vi "_Get Measurement.vi"(8 "error in (no error)":errorcluster, 10 "Command":string, 11 "VISA resource name":refnum<visa-resource-name>) -> (0 "error out":errorcluster, 1 "Data":dbl[](array[numeric]) format="%^.3e", 2 "Reliability":i32, 3 "VISA resource name out":refnum<visa-resource-name>)   [LabVIEW 2020, in "Rohde&Schwarz CMXP GPRF.lvlib"]
uses:
  <instrlib>/Rohde&Schwarz CMXP GPRF/Rohde&Schwarz CMXP GPRF.lvlib
  <instrlib>/Rohde&Schwarz CMXP GPRF/Private/rsidr_core.llb/rsidr_core.lvlib
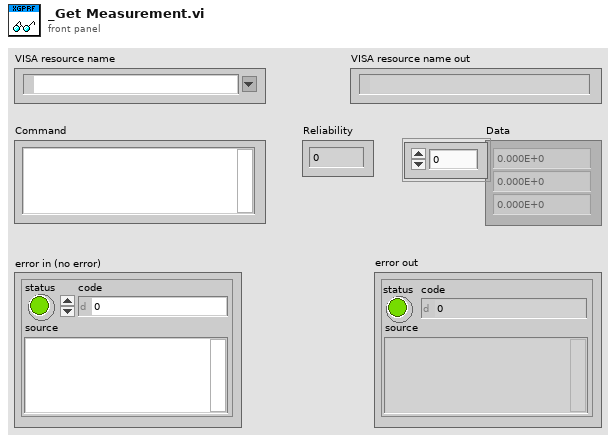
[diagram p1: front panel]
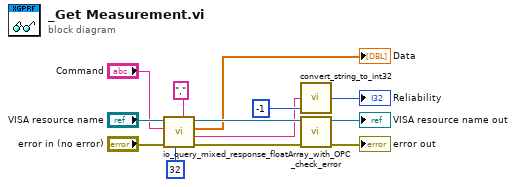
[diagram p0: block diagram]
diagram:
  n1 = call <instrlib>:"io_query_mixed_response_floatArray_with_OPC.vi"("Ascii part splitter"=",", "Ascii part max length"=32, "error in"="error in (no error)", "Query"="Command", "VISA resource name"="VISA resource name") -> ("error out"=w11:errorcluster, "ASCII part out"=w1:string, "Numbers out"=→"Data":dbl[], "VISA resource name out"=w10:refnum<visa-resource-name>)  [unwired: 3 in]
  n2 = call <instrlib>:"convert_string_to_int32.vi"("default (0)"=-1, "String in"=w1) -> ("int32 value out"=→"Reliability":i32)  [unwired: 3 in]
  n3 = call <instrlib>:"_check_error.vi"("error in (no error)"=w11, "VISA resource name"=w10) -> ("error out"=→"error out":errorcluster, "VISA resource name out"=→"VISA resource name out":refnum<visa-resource-name>)  [unwired: 8 in]
